vi "RecipeUpdateVariables.vi"(6 "Index_List":i32[](array[numeric]), 8 "error in (no error)":errorcluster, 10 "Recipe_Input":string[][](array[string]), 11 "DeviceSetup":variant[](array[variant])) -> (0 "error out":errorcluster, 3 "DeviceSetup_Update":variant[](array[variant]))   [LabVIEW 2014]
uses:
  Config_RFSA_Spectrum_Acq.ctl
  Config_RFSA_IQ_Acq.ctl
  Config_RFSA_Vertical.ctl
  Config_RFSG.ctl
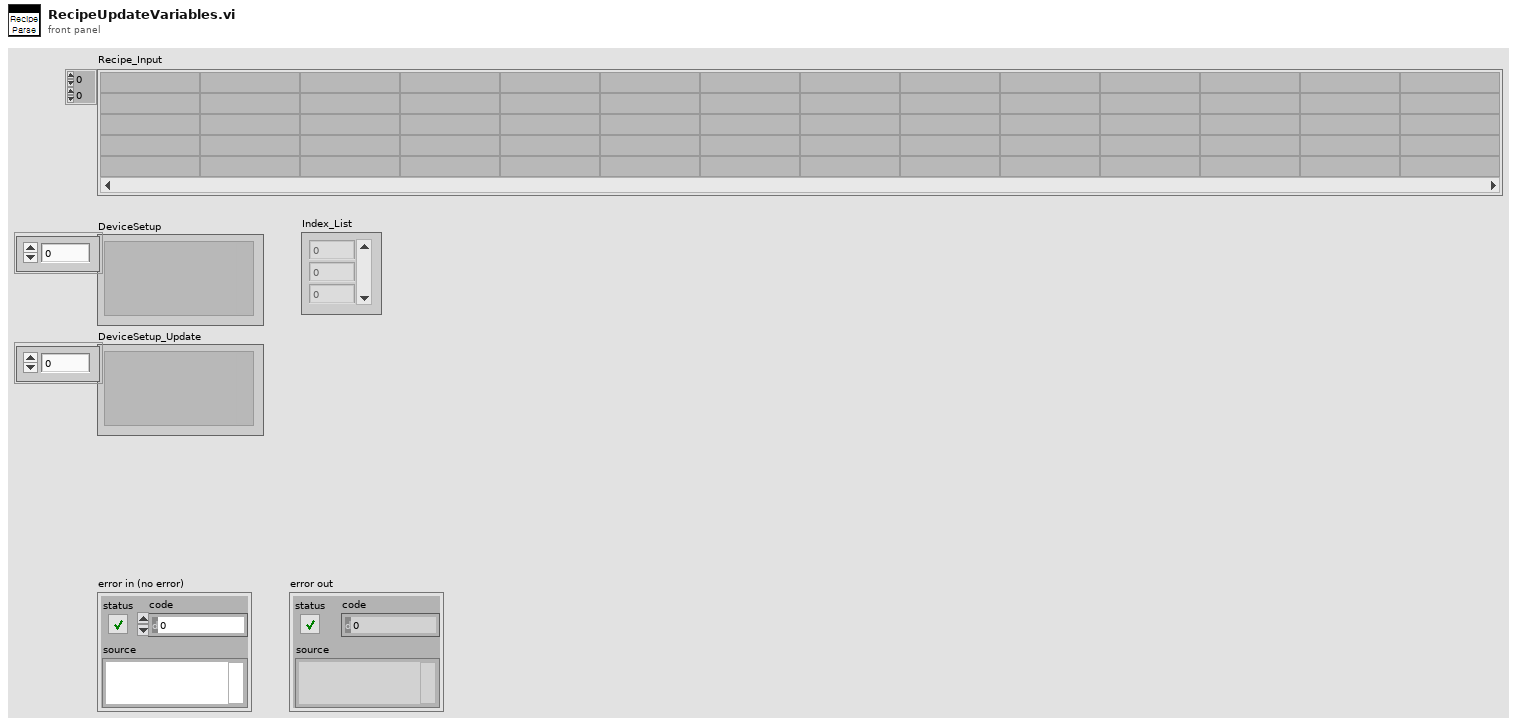
[diagram p1: front panel]
types:
  T1 = typedef "Config_RFSG.ctl" = cluster{"Carrier Frequency":dbl, "RF Power Level (dBm)":dbl, "SG External Gain (dBm)":dbl, "Standard":enum16{"LTE", "WCDMA", "GSM", "EDGE", "CW", "CWM"}}
  T2 = typedef "Config_RFSA_Vertical.ctl" = cluster{"Acquisition Type":i32, "Reference Level (dBm)":dbl, "External Gain (dB)":dbl}
  T3 = typedef "Config_RFSA_IQ_Acq.ctl" = cluster{"carrier frequency":dbl, "IQ rate (S/s)":dbl, "samples per record":i64}
  T4 = typedef "Config_RFSA_Spectrum_Acq.ctl" = cluster{"Resolution Bandwidth (Hz)":dbl, "Start Frequency (Hz)":dbl, "Stop Frequency (Hz)":dbl}
  T5 = enum16{"LTE", "WCDMA", "GSM", "EDGE", "CW", "CWM"}
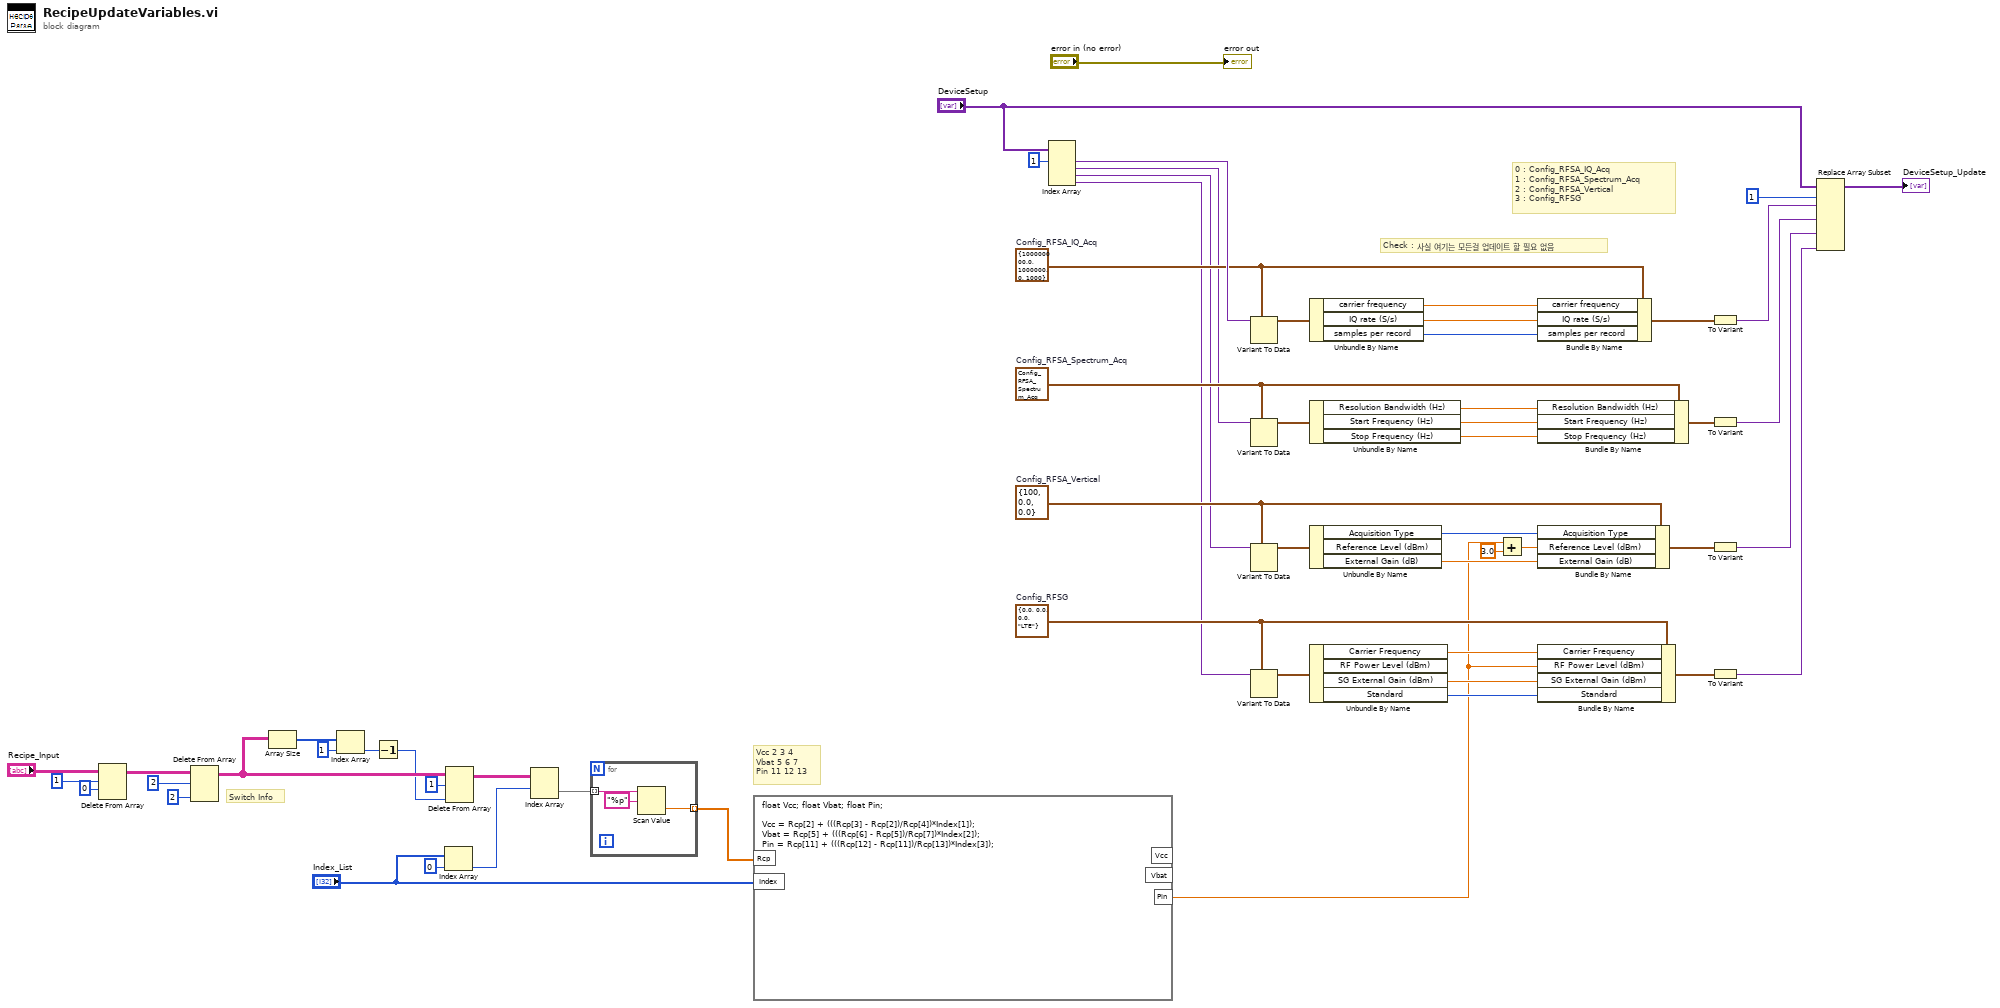
[diagram p0: block diagram]
diagram:
  w31 = T1 {"Carrier Frequency"=0.0, "RF Power Level (dBm)"=0.0, "SG External Gain (dBm)"=0.0, "Standard"=enum."LTE"}  # Config_RFSG
  w35 = T2 {"Acquisition Type"=100, "Reference Level (dBm)"=0.0, "External Gain (dB)"=0.0}  # Config_RFSA_Vertical
  w43 = T3 {"carrier frequency"=100000000.0, "IQ rate (S/s)"=1000000.0, "samples per record"=1000}  # Config_RFSA_IQ_Acq
  w37 = T4 {"Resolution Bandwidth (Hz)"=10000.0, "Start Frequency (Hz)"=90000000.0, "Stop Frequency (Hz)"=110000000.0}  # Config_RFSA_Spectrum_Acq
  # "Check : 사실 여기는 모든걸 업데이트 할 필요 없음"
  # "Vcc 2 3 4\nVbat 5 6 7\nPin 11 12 13"
  # "Switch Info"
  # "0 : Config_RFSA_IQ_Acq\n1 : Config_RFSA_Spectrum_Acq\n2 : Config_RFSA_Vertical\n3 : Config_RFSG"
  n1 = Delete From Array(array="Recipe_Input", length=1, index (row)=0) -> (array with subset deleted=w21:string[][])  [unwired: 1 in, 1 out]
  n2 = Delete From Array(array=w21, length=2, index (col)=2 ("disabled index (col)")) -> (array with subset deleted=w16:string[][])  [unwired: 1 in, 1 out]
  n3 = Array Size(array=w16) -> (size(s)=w18:i32[])
  n4 = Index Array(array=w18, index=1) -> (element=w15:i32)
  n5 = Decrement(x=w15) -> (x-1=w13:i32)
  n6 = Index Array(array="Index_List", index=0) -> (element=w7:i32)
  n7 = Delete From Array(array=w16, length=1, index (col)=w13) -> (array with subset deleted=w12:string[][])  [unwired: 1 in, 1 out]
  n8 = Index Array(array=w12, index (row)=w7) -> (element=w11:string[])  [unwired: 1 in]
  n9 = for {
    tunnel: w11 -> [w60] mode=indexing
    tunnel: [w58] -> w6 mode=indexing
    n10 = Scan Value(string=w60, format string="%p") -> (value=w58:dbl)  [unwired: 1 in, 1 out]
  }
  n11 = formula code="float Vcc; float Vbat; float Pin;\n\nVcc = Rcp[2] + (((Rcp[3] - Rcp[2])/Rcp[4])*Index[1]);\nVbat = Rcp[5] + (((Rcp[6] - Rcp[5])/Rcp[7])*Index[2]); \nPin = Rcp[11] + (((Rcp[12] - Rcp[11])/Rcp[13])*Index[3]);"("Index"="Index_List", "Rcp"=w6) -> ("Pin"=w5:dbl)  [unwired: 2 out]
  n12 = Index Array(array="DeviceSetup", index #1=1 ("index")) -> (element #1=w44:variant, element #2=w26:variant, element #3=w25:variant, element #4=w24:variant)  [unwired: 3 in]
  n13 = Variant To Data(type=w43, Variant=w44) -> (data=w42:T3)  [unwired: 1 in, 1 out]
  n14 = Variant To Data(type=w37, Variant=w26) -> (data=w36:T4)  [unwired: 1 in, 1 out]
  n15 = Variant To Data(type=w35, Variant=w25) -> (data=w34:T2)  [unwired: 1 in, 1 out]
  n16 = Variant To Data(type=w31, Variant=w24) -> (data=w30:T1)  [unwired: 1 in, 1 out]
  n17 = Unbundle By Name(w42) -> ("carrier frequency"=w41:dbl, "IQ rate (S/s)"=w40:dbl, "samples per record"=w39:i64)
  n18 = Unbundle By Name(w36) -> ("Resolution Bandwidth (Hz)"=w38:dbl, "Start Frequency (Hz)"=w2:dbl, "Stop Frequency (Hz)"=w1:dbl)
  n19 = Unbundle By Name(w34) -> ("Acquisition Type"=w33:i32, "External Gain (dB)"=w32:dbl)  [unwired: 1 out]
  n20 = Unbundle By Name(w30) -> ("Carrier Frequency"=w29:dbl, "SG External Gain (dBm)"=w28:dbl, "Standard"=w27:T5)  [unwired: 1 out]
  n21 = Add(x=w5, y=3.0) -> (x+y=w3:dbl)
  n22 = Bundle By Name(cluster=w43, "carrier frequency"=w41, "IQ rate (S/s)"=w40, "samples per record"=w39) -> (w57:T3)
  n23 = Bundle By Name(cluster=w37, "Resolution Bandwidth (Hz)"=w38, "Start Frequency (Hz)"=w2, "Stop Frequency (Hz)"=w1) -> (w56:T4)
  n24 = Bundle By Name(cluster=w35, "Acquisition Type"=w33, "Reference Level (dBm)"=w3, "External Gain (dB)"=w32) -> (w55:T2)
  n25 = Bundle By Name(cluster=w31, "Carrier Frequency"=w29, "RF Power Level (dBm)"=w5, "SG External Gain (dBm)"=w28, "Standard"=w27) -> (w54:T1)
  n26 = To Variant(anything=w57) -> (Variant=w52:variant)
  n27 = To Variant(anything=w56) -> (Variant=w51:variant)
  n28 = To Variant(anything=w55) -> (Variant=w50:variant)
  n29 = To Variant(anything=w54) -> (Variant=w49:variant)
  n30 = Replace Array Subset(array="DeviceSetup", new element #1=w52, index #1=1 ("index"), new element #2=w51, new element #3=w50, new element #4=w49) -> (→"DeviceSetup_Update":variant[])  [unwired: 3 in]
  "error out" <- "error in (no error)"
